vi "Array offset with truncation.vi"(8 "New starting value":dbl, 9 "Truncate up":bool, 11 "Input array":dbl[](array[numeric])) -> (1 "Truncated array with new starting value":dbl[](array[numeric]), 3 "Array with new starting value":dbl[](array[numeric]))   [LabVIEW 2018]
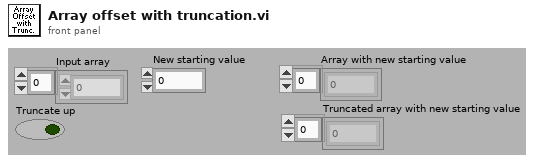
[diagram p1: front panel]
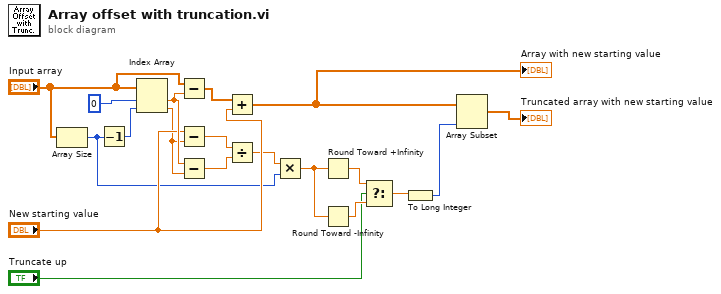
[diagram p0: block diagram]
diagram:
  n1 = Array Size(array="Input array") -> (size(s)=w9:i32)
  n2 = Decrement(x=w9) -> (x-1=w16:i32)
  n3 = Index Array(array="Input array", index #1=0 ("index"), index #2=w16) -> (element #1=w15:dbl, element #2=w13:dbl)
  n4 = Subtract(x="Input array", y=w15) -> (x-y=w18:dbl[])
  n5 = Subtract(x="New starting value", y=w13) -> (x-y=w12:dbl)
  n6 = Subtract(x=w15, y=w13) -> (x-y=w11:dbl)
  n7 = Add(x=w18, y="New starting value") -> (x+y=w7:dbl[])
  "Array with new starting value" <- w7
  n8 = Divide(x=w12, y=w11) -> (x/y=w10:dbl)
  n9 = Multiply(x=w10, y=w9) -> (x*y=w5:dbl)
  n10 = Round Toward +Infinity(x=w5) -> (ceil(x): smallest int >= x=w2:dbl)
  n11 = Round Toward -Infinity(1:w5) -> (0:w4:dbl)
  n12 = Select(t=w2, s="Truncate up", f=w4) -> (s? t:f=w3:dbl)
  n13 = To Long Integer(number=w3) -> (32bit integer=w8:i32)
  n14 = Array Subset(array=w7, length=w8) -> (→"Truncated array with new starting value":dbl[])  [unwired: 1 in]
